vi "SeCrTS-DD NS Receiver.vi"(11 "NOT DIS Out":T1) -> ()   [LabVIEW 2022 SP3]
uses:
  Control/SeCrTS-Notifier Ref.ctl
  Globals/SeCrTS-DD globals.vi
  <resource>/objmgr/ni.dex.rc
panel:
  out "timed out?":bool
  out "x":u32
  out "error out":errorcluster
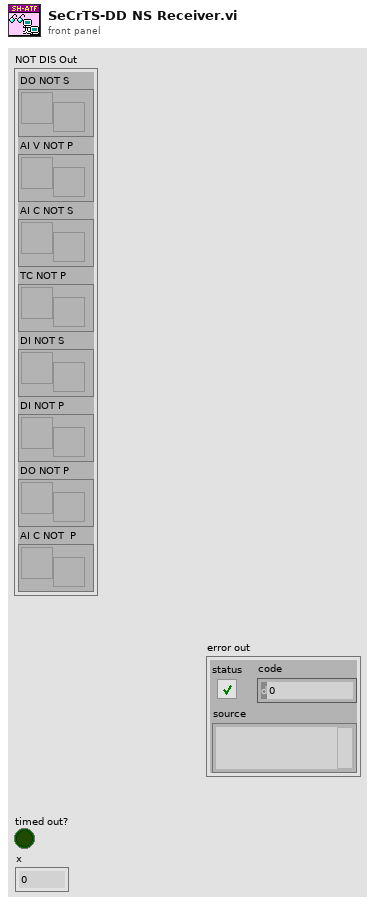
[diagram p1: front panel]
types:
  T1 = typedef "SeCrTS-Notifier Ref.ctl" = cluster{"DO NOT S":refnum<notifier>, "AI V NOT P":refnum<notifier>, "AI C NOT S":refnum<notifier>, "TC NOT P":refnum<notifier>, "DI NOT S":refnum<notifier>, "DI NOT P":refnum<notifier>, "DO NOT P":refnum<notifier>, "AI C NOT  P":refnum<notifier>}
  T2 = cluster{"In Progress":bool, "reader url":refnum<k21>}
  T3 = enum16{"Initialize", "Wait for connection", "Send data", "Exit", "Receive Data"}
  T4 = cluster{"AI_V_Data":waveform(dbl)[][], "AI_C_Data":waveform(dbl)[][], "AO_Data":waveform(dbl)[][], "DO_Data":waveform(dbl)[][], "DI_Data":digitalwaveform[][], "ACC_Data":waveform(dbl)[][], "TC Data":waveform(dbl)[][], "Drive_A_C":waveform(dbl)[][], "Drive_A_D":waveform(dbl)[][], "Drive_L_C":waveform(dbl)[][], "Drive_L_D":waveform(dbl)[][], "RT Time":timestamp}
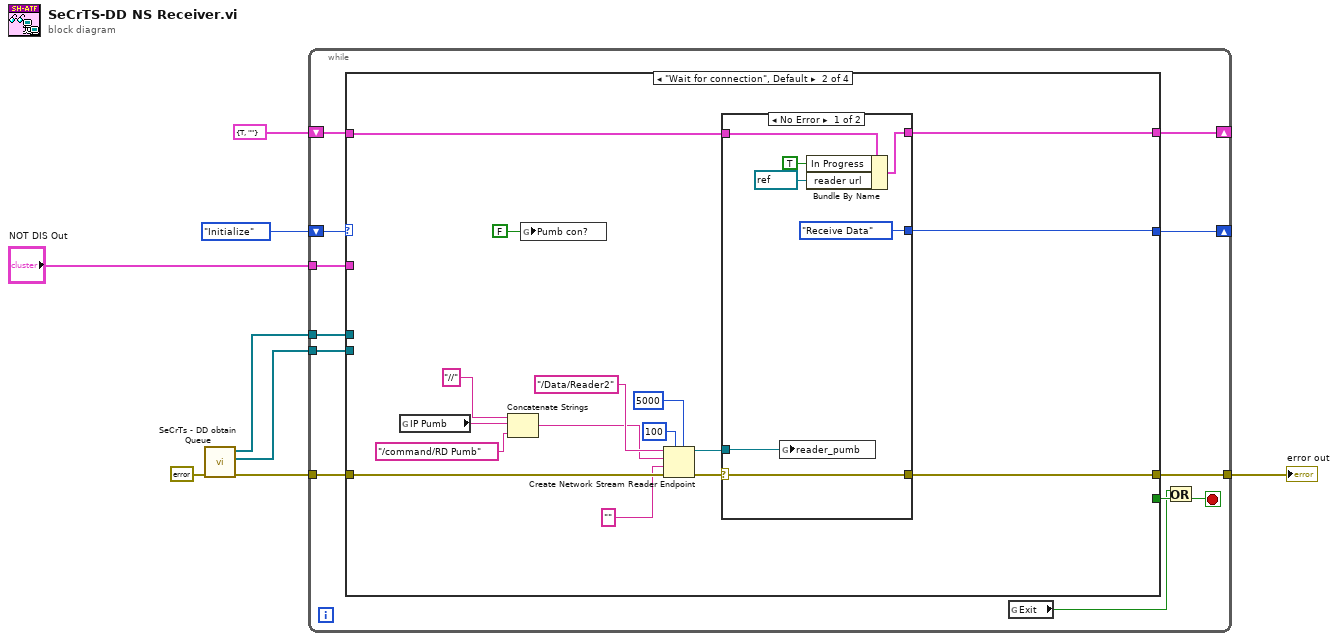
[diagram p0: block diagram]
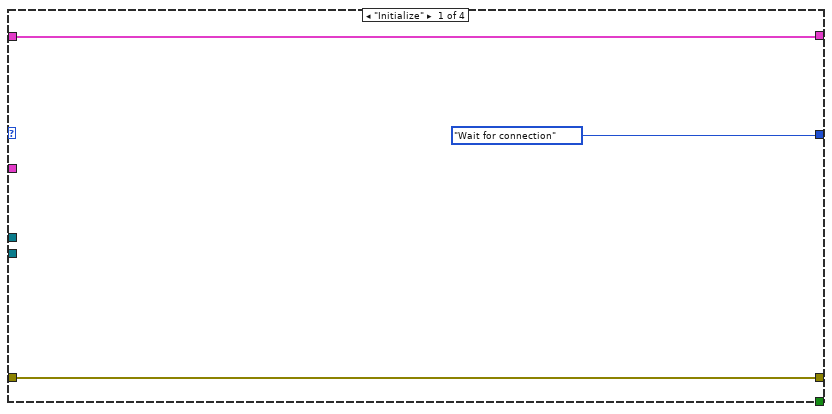
[diagram p2: hidden frame]
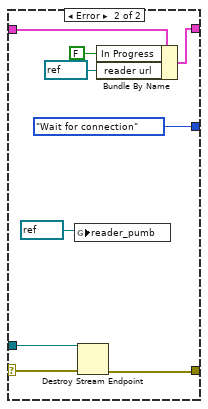
[diagram p3: hidden frame]
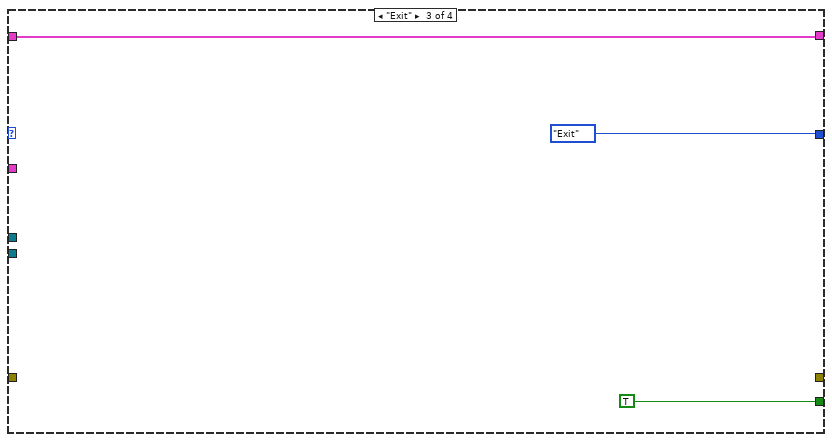
[diagram p4: hidden frame]
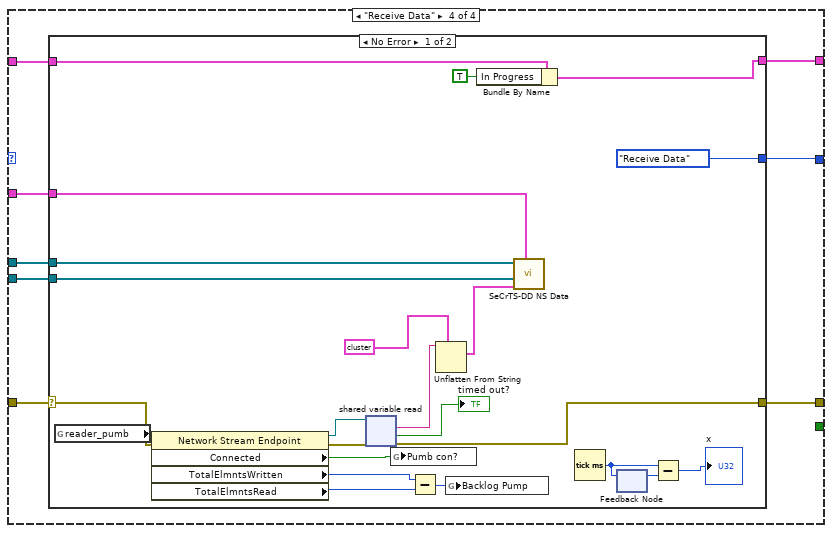
[diagram p5: hidden frame]
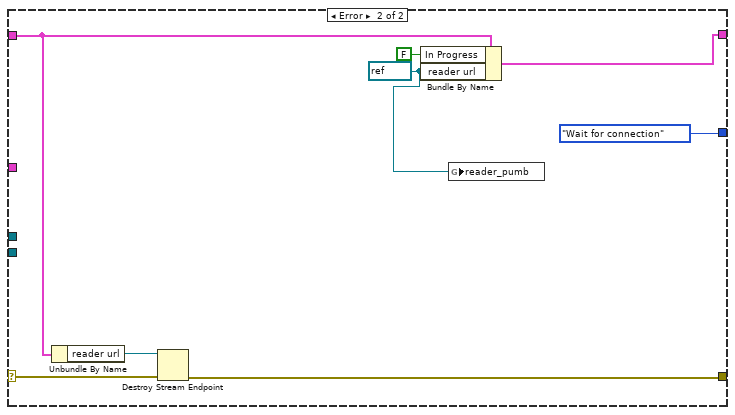
[diagram p6: hidden frame]
diagram:
  n1 = call "SeCrTs - DD obtain Queue.vi"("error in"=errorcluster {"status"=FALSE, "code"=0, "source"=""}) -> ("error out"=w5:errorcluster, "AI_V_Data P\nAI_C_Data P\nAO_Data P\nDO_Data P\nACC_Data P\nTC Data P\nDrive_A_C \nDrive_A_D\nAI_C_Data S\nDO_Data S"=w3:refnum<queue>[], "DI P\nDI S"=w4:refnum<queue>[])  [unwired: 8 in]
  n2 = while {
    shift-right: [w18] -> _
    shift-left: T3."Initialize" -> [w20]
    shift-right: [w16] -> _
    shift-left: T2 {"In Progress"=TRUE, "reader url"=""} -> [w17]
    tunnel: w5 -> [w15]
    tunnel: [w14] -> w6
    tunnel: "NOT DIS Out" -> [w11]
    tunnel: w4 -> [w10]
    tunnel: w3 -> [w9]
    stop <- w13 stop-if-true
    n3 = case shown="\"Wait for connection\", Default" w20 {
      tunnel: [_ _ TRUE _] -> w19
      tunnel: [T3."Wait for connection" w35 T3."Exit" w63] -> w18
      tunnel: w17 -> [w23 w39 w57 w66]
      tunnel: [w23 w38 w57 w64] -> w16
      tunnel: w15 -> [w21 w37 _ w65]
      tunnel: [w21 w36 _ w62] -> w14
      tunnel: w11 -> [_ _ _ w61]
      tunnel: w10 -> [_ _ _ w60]
      tunnel: w9 -> [_ _ _ w59]
      frame "Initialize" {
      }
      frame "Wait for connection", Default {
        n4 = global read "SeCrTS-DD globals.vi" "IP Pumb"() -> (w26:string)
        n5 = Concatenate Strings("//" ("string"), w26, "/command/RD Pumb" ("reader url")) -> (w28:string)
        n6 = global write "SeCrTS-DD globals.vi" "Pumb con?"(FALSE ("Storage con?")) -> ()
        n7 = Create Network Stream Reader Endpoint(5:5000 ("timeout in ms (-1)"), 7:100 ("reader buffer size"), 8:w37, 9:"", 10:w28, 11:"/Data/Reader2" ("writer name")) -> (0:w32:errorcluster, 3:w33:refnum<k21>)  [unwired: 1 in]
        n8 = case shown="No Error" w32 {
          selector: w32 -> [w43 w51]
          tunnel: w39 -> [w46 w55]
          tunnel: w33 -> [w41 w52]
          tunnel: [w44 w54] -> w38
          tunnel: [w43 w50] -> w36
          tunnel: [T3."Receive Data" T3."Wait for connection"] -> w35
          frame No Error {
            n9 = global write "SeCrTS-DD globals.vi" "reader_pumb"(w41) -> ()
            n10 = Bundle By Name(cluster=w46, "In Progress"=TRUE, "reader url"=refnum<k21> refnum) -> (w44:T2)
          }
          frame Error {
            n11 = global write "SeCrTS-DD globals.vi" "reader_pumb"(refnum<k21> refnum ("reader")) -> ()
            n12 = Destroy Stream Endpoint(8:w51, 11:w52) -> (0:w50:errorcluster)
            n13 = Bundle By Name(cluster=w55, "In Progress"=FALSE, "reader url"=refnum<k21> refnum) -> (w54:T2)
          }
        }
      }
      frame "Exit" {
      }
      frame "Receive Data" {
        n14 = case shown="No Error" w65 {
          selector: w65 -> [w84 w92]
          tunnel: w66 -> [w89 w95]
          tunnel: [w88 w97] -> w64
          tunnel: [T3."Receive Data" T3."Wait for connection"] -> w63
          tunnel: [w81 w91] -> w62
          tunnel: w61 -> [w74 _]
          tunnel: w60 -> [w73 _]
          tunnel: w59 -> [w72 _]
          frame No Error {
            n15 = global read "SeCrTS-DD globals.vi" "reader_pumb"() -> (w82:refnum<k21>)
            n16 = property class="Network Stream Endpoint"(reference=w82, error in=w84) -> (reference out=w86:refnum<k21>, error out=w83:errorcluster, "Connected"=w80:bool, "TotalElmntsWritten"=w69:u64, "TotalElmntsRead"=w68:u64)
            n17 = shared-variable-read(w86, w83) -> (w81:errorcluster, →"timed out?":bool, w76:string)  [unwired: 1 in, 1 out]
            n18 = global write "SeCrTS-DD globals.vi" "Pumb con?"(w80) -> ()
            n19 = Subtract(x=w69, y=w68) -> (x-y=w67:u64)
            n20 = Unflatten From String(type=T4 data[101864B] ("data out"), binary string=w76) -> (value=w70:T4)  [unwired: 3 in, 2 out]
            n21 = global write "SeCrTS-DD globals.vi" "Backlog Pump"(w67) -> ()
            n22 = Bundle By Name(cluster=w89, "In Progress"=TRUE) -> (w88:T2)
            n23 = call "SeCrTS-DD NS Data.vi"("NOT DIS Out"=w74, "value"=w70, "AI_V_Data P\nAI_C_Data P\nAO_Data P\nDO_Data P\nACC_Data P\nTC Data P\nDrive_A_C \nDrive_A_D\nAI_C_Data S\nDO_Data S"=w72, "DI P\nDI S"=w73) -> ()  [unwired: 8 in]
            n24 = Tick Count (ms)() -> (millisecond timer value=w78:u32)
            n25 = feedback-in #1(w78) -> ()
            n26 = feedback #1() -> (w79:u32)  [unwired: 1 in]
            n27 = Subtract(x=w78, y=w79) -> (x-y=→"x":u32)
          }
          frame Error {
            w90 = refnum<k21> refnum ("reader url")
            n28 = Unbundle By Name(w95) -> ("reader url"=w94:refnum<k21>)
            n29 = Destroy Stream Endpoint(8:w92, 11:w94) -> (0:w91:errorcluster)
            n30 = Bundle By Name(cluster=w95, "In Progress"=FALSE, "reader url"=w90) -> (w97:T2)
            n31 = global write "SeCrTS-DD globals.vi" "reader_pumb"(w90) -> ()
          }
        }
      }
    }
    n32 = global read "SeCrTS-DD globals.vi" "Exit"() -> (w12:bool)
    n33 = Or(x=w12, y=w19) -> (x .or. y?=w13:bool)
  }
  "error out" <- w6
